vi "Generate Service Name.vi"(8 "error in (no error)":errorcluster, 9 "Bitness Text":string, 10 "LV Version":string, 11 "VI Path":path) -> (0 "error out":errorcluster, 3 "Service Name":string)   [LabVIEW 2015, in "CLI.lvclass"]
uses:
  CLI.lvclass
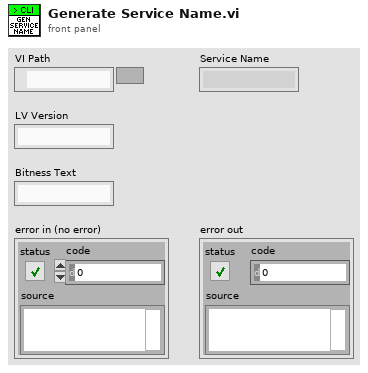
[diagram p1: front panel]
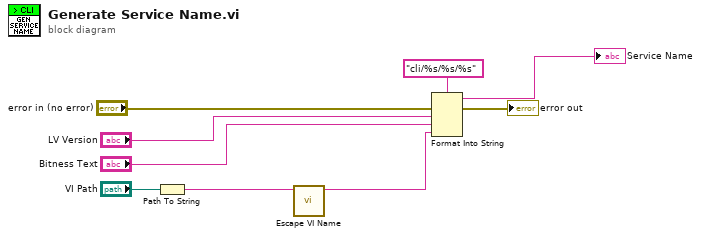
[diagram p0: block diagram]
diagram:
  n1 = Path To String(path="VI Path") -> (string=w9:string)
  n2 = call "Escape VI Name.vi"("Path"=w9) -> ("Escaped"=w1:string)  [unwired: 10 in]
  n3 = Format Into String(format string="cli/%s/%s/%s", error in="error in (no error)", "LV Version", "Bitness Text", w1) -> (resulting string=→"Service Name":string, error out=→"error out":errorcluster)  [unwired: 1 in]
